vi "Reset Count (Serial Bus - CAN).vi"(8 "error in (no error)":errorcluster, 10 "Serial Bus Name (1: Serial Bus 1)":i32(ring)=1 items=["Serial Bus 1"=1, "Serial Bus 2"=2], 11 "VISA resource name":refnum<visa-resource-name>) -> (0 "error out":errorcluster, 3 "VISA resource name out":refnum<visa-resource-name>)   [LabVIEW 2015, in "Agilent 2000 3000 X-Series.lvlib"]
doc: "Resets the CAN frame counters."
uses:
  Agilent 2000 3000 X-Series.lvlib
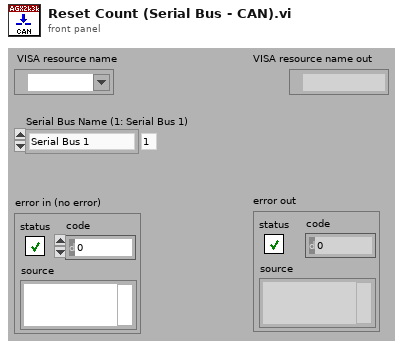
[diagram p1: front panel]
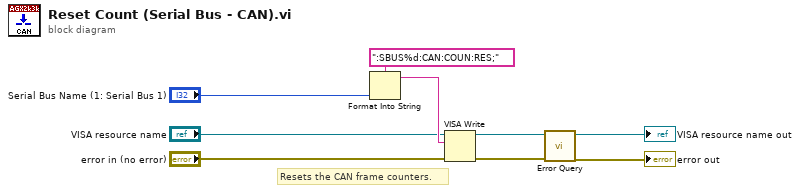
[diagram p0: block diagram]
diagram:
  # "Resets the CAN frame counters."
  n1 = Format Into String(format string=":SBUS%d:CAN:COUN:RES;", "Serial Bus Name (1: Serial Bus 1)") -> (resulting string=w7:string)  [unwired: 2 in, 1 out]
  n2 = VISA Write(VISA resource name="VISA resource name", write buffer=w7, error in (no error)="error in (no error)") -> (VISA resource name out=w4:refnum<visa-resource-name>, error out=w3:errorcluster)  [unwired: 1 out]
  n3 = call "Error Query.vi"("error in (no error)"=w3, "VISA resource name"=w4) -> ("error out"=→"error out":errorcluster, "VISA resource name out"=→"VISA resource name out":refnum<visa-resource-name>)  [unwired: 8 out]
